vi "Data Server Decode Command.vi"(5 "Corrector names":string[](array[string])=["ACH01B", "ACH02", "ACH03B", "ACH04", "ACH05A", "ACH06", "ACH07A", "ACH07B", "ACH08"], 7 "BPM names":string[](array[string])=["ACH01B", "ACH02", "ACH03B", "ACH04", "ACH05A", "ACH06", "ACH07A", "ACH07B", "ACH08"], 8 "error in (no error)":errorcluster, 11 "Input string":string) -> (0 "error out":errorcluster, 1 "BPM and PS index":T1, 2 "Number of samples":u32, 4 "Stop Acquisition?":bool)   [LabVIEW 2011, in "Data Server VIs.lvlib"]
uses:
  Data Server VIs.lvlib
  Types Definitions/Type BPM and PS select cluster.ctl
  Type Definitions.lvlib
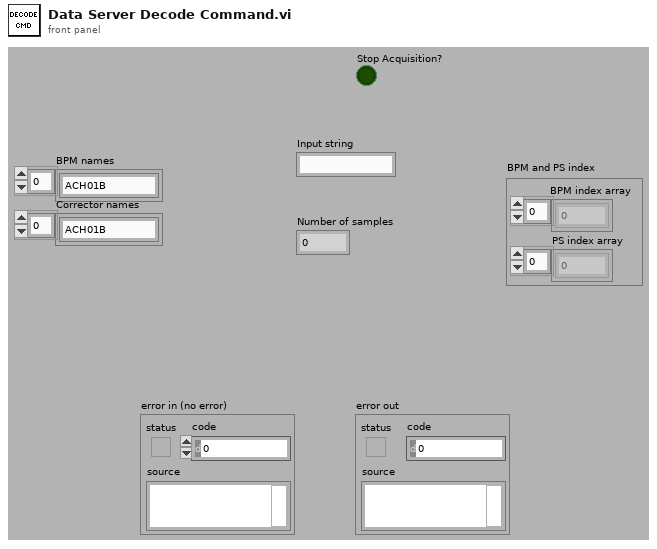
[diagram p1: front panel]
types:
  T1 = typedef "Type Definitions.lvlib/Type BPM and PS select cluster.ctl" = cluster{"BPM index array":u32[], "PS index array ":u32[]}
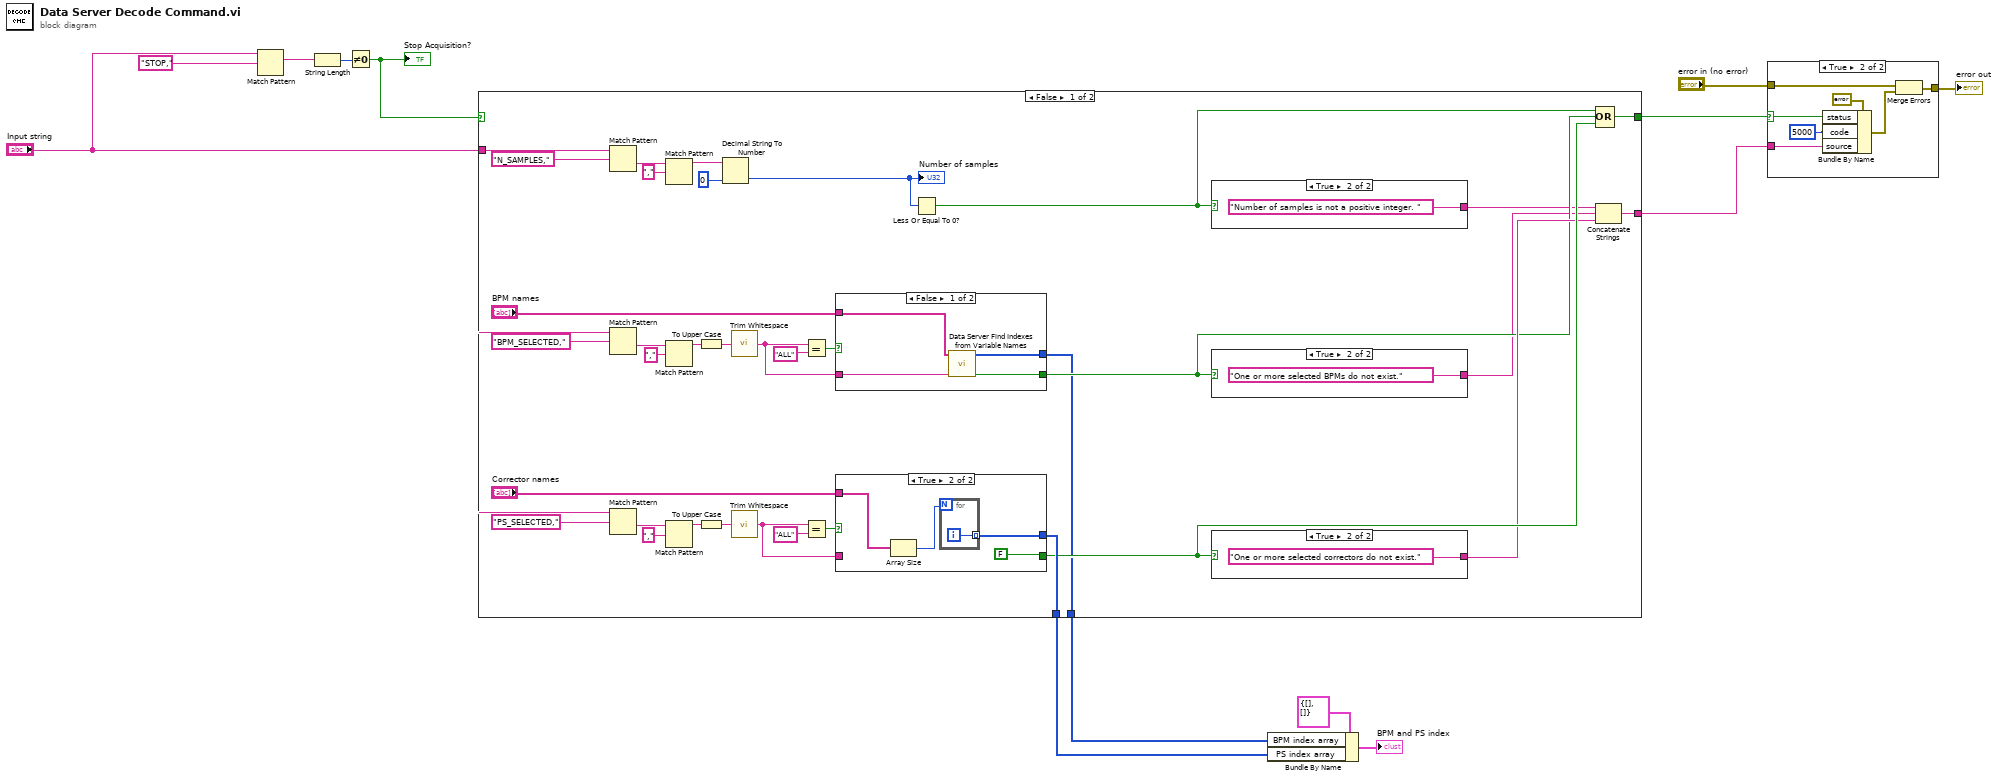
[diagram p0: block diagram]
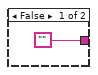
[diagram p2: hidden frame]
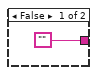
[diagram p3: hidden frame]
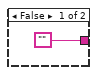
[diagram p4: hidden frame]
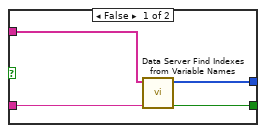
[diagram p5: hidden frame]
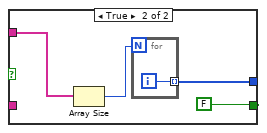
[diagram p6: hidden frame]
diagram:
  n1 = Match Pattern(string="Input string", regular expression="STOP,") -> (match substring=w5:string)  [unwired: 1 in, 3 out]
  n2 = String Length(string=w5) -> (length=w4:i32)
  n3 = Not Equal To 0?(x=w4) -> (x != 0?=w3:bool)
  "Stop Acquisition?" <- w3
  n4 = case shown="False" w3 {
    tunnel: [w28 _] -> w11
    tunnel: [w25 _] -> w1
    tunnel: [w18 _] -> w8
    tunnel: [w17 _] -> w2
    tunnel: "Input string" -> [w15 _]
    frame False {
      n5 = Match Pattern(string=w15, regular expression="N_SAMPLES,") -> (after substring=w47:string)  [unwired: 1 in, 3 out]
      n6 = Match Pattern(string=w15, regular expression="BPM_SELECTED,") -> (after substring=w41:string)  [unwired: 1 in, 3 out]
      n7 = Match Pattern(string=w15, regular expression="PS_SELECTED,") -> (after substring=w31:string)  [unwired: 1 in, 3 out]
      n8 = Match Pattern(string=w47, regular expression=",") -> (before substring=w45:string)  [unwired: 1 in, 3 out]
      n9 = Match Pattern(string=w41, regular expression=",") -> (before substring=w29:string)  [unwired: 1 in, 3 out]
      n10 = Match Pattern(string=w31, regular expression=",") -> (before substring=w33:string)  [unwired: 1 in, 3 out]
      n11 = To Upper Case(1:w29) -> (0:w38:string)
      n12 = To Upper Case(1:w33) -> (0:w35:string)
      n13 = Decimal String To Number(string=w45, default (0L)=u32 0 ("y")) -> (number=w43:u32)  [unwired: 1 in, 1 out]
      "Number of samples" <- w43
      n14 = call <vilib>:"Trim Whitespace.vi"("string"=w38) -> ("trimmed string"=w36:string)  [unwired: 1 in]
      n15 = call <vilib>:"Trim Whitespace.vi"("string"=w35) -> ("trimmed string"=w27:string)  [unwired: 1 in]
      n16 = Equal?(x=w36, y="ALL") -> (x = y?=w37:bool)
      n17 = Equal?(x=w27, y="ALL") -> (x = y?=w26:bool)
      n18 = case shown="False" w37 {
        tunnel: w36 -> [w67 _]
        tunnel: [w65 w68] -> w17
        tunnel: [w64 FALSE ("Index Fault")] -> w22
        tunnel: "BPM names" -> [w66 w69]
        frame False {
          n19 = call "Data Server Find Indexes from Variable Names.vi"("Comand string"=w67, "Variable names"=w66) -> ("Command error"=w64:bool, "Index array"=w65:i32[])  [unwired: 8 in]
        }
        frame True {
          n20 = Array Size(array=w69) -> (size(s)=w70:i32)
          n21 = for {
            N: w70 -> [_]
            tunnel: [w72] -> w68 mode=indexing
            i -> [w72]
          }
        }
      }
      n22 = case shown="True" w26 {
        tunnel: w27 -> [w56 _]
        tunnel: [w57 w59] -> w25
        tunnel: [w55 FALSE ("Index Fault")] -> w24
        tunnel: "Corrector names" -> [w58 w60]
        frame False {
          n23 = call "Data Server Find Indexes from Variable Names.vi"("Comand string"=w56, "Variable names"=w58) -> ("Command error"=w55:bool, "Index array"=w57:i32[])  [unwired: 8 in]
        }
        frame True {
          n24 = Array Size(array=w60) -> (size(s)=w61:i32)
          n25 = for {
            N: w61 -> [_]
            tunnel: [w63] -> w59 mode=indexing
            i -> [w63]
          }
        }
      }
      n26 = Less Or Equal To 0?(x=w43) -> (x <= 0?=w21:bool)
      n27 = case shown="True" w21 {
        tunnel: ["" "Number of samples is not a positive integer. "] -> w20
        frame False {
        }
        frame True {
        }
      }
      n28 = case shown="True" w22 {
        tunnel: ["" "One or more selected BPMs do not exist."] -> w19
        frame False {
        }
        frame True {
        }
      }
      n29 = case shown="True" w24 {
        tunnel: ["" "One or more selected correctors do not exist."] -> w23
        frame False {
        }
        frame True {
        }
      }
      n30 = Compound Arithmetic op=OR(w21, w22, w24) -> (w28:bool)
      n31 = Concatenate Strings(w20, w19, w23) -> (w18:string)
    }
    frame True {
    }
  }
  n32 = Bundle By Name(cluster=T1 {"BPM index array"=[], "PS index array "=[]} ("Cluster"), "BPM index array"=w2, "PS index array"=w1) -> (→"BPM and PS index":T1)
  n33 = case shown="True" w11 {
    selector: w11 -> [_ w74]
    tunnel: "error in (no error)" -> [w73 w78]
    tunnel: [w73 w76] -> w12
    tunnel: w8 -> [_ w75]
    frame False {
    }
    frame True {
      n34 = Bundle By Name(cluster=errorcluster {"status"=TRUE, "code"=0, "source"=""} ("error out"), "status"=w74, "code"=5000, "source"=w75) -> (w77:errorcluster)
      n35 = Merge Errors(w78, w77) -> (w76:errorcluster)
    }
  }
  "error out" <- w12
